vi "Get Maximum Exposure.vi"(11 "MaxExp":sgl) -> (2 "function return":u32, 3 "MaxExp out":sgl)   [LabVIEW 2018, in "Copy of Andor SDK.lvlib"]
doc: "EXPNETTYPE unsigned int WINAPI GetMaximumExposure(float * MaxExp);"
uses:
  Copy of Andor SDK.lvlib
  <userlib>/Andor SDK/ATMCD32D.dll
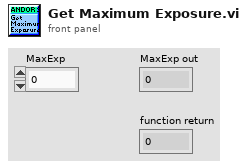
[diagram p1: front panel]
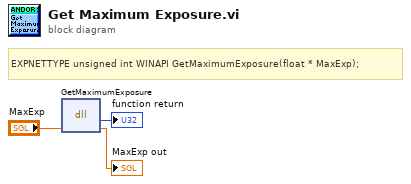
[diagram p0: block diagram]
diagram:
  # "EXPNETTYPE unsigned int WINAPI GetMaximumExposure(float * MaxExp);"
  n1 = dll-call lib="C:/Program Files (x86)/National Instruments/LabVIEW 2018/user.lib/Andor SDK/ATMCD32D.*" fn="GetMaximumExposure"("MaxExp"="MaxExp") -> (→"function return":u32, "MaxExp"=→"MaxExp out":sgl)  [unwired: 3 in, 2 out]
